vi "Return Msg.vi"(8 "error in (no error)":errorcluster, 11 "Add Control_Behavior.lvclass":refnum<class "Add Control_Behavior.lvclass">) -> (0 "error out":errorcluster, 2 "Console Reply.lvclass":refnum<class "Console Reply.lvclass">, 3 "Panel Behavior.lvclass":refnum<class "Panel Behavior.lvclass">)   [LabVIEW 2015, in "Add Control_Behavior.lvclass"]
uses:
  Add Control_Behavior.lvclass
  _Depences/Panel API/Panel Request/Panle Requeset Behavior/Panel Behavior.lvclass
  _Depences/Panel API/Console Reply/Console Reply/Console Reply.lvclass
  Console Reply Add Control Result/Console Reply Add Control.lvclass
  Add Control_Behavior.lvclass/Add Control_Behavior.ctl
  Console Reply Add Control Result/Console Reply Add Control.lvclass/Console Reply Add Control.ctl
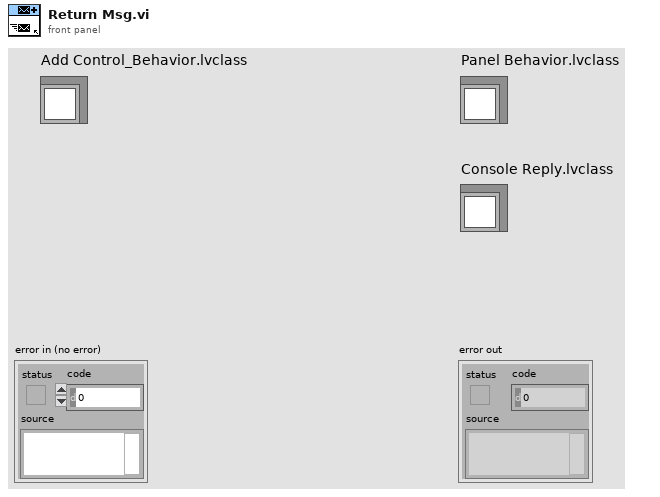
[diagram p1: front panel]
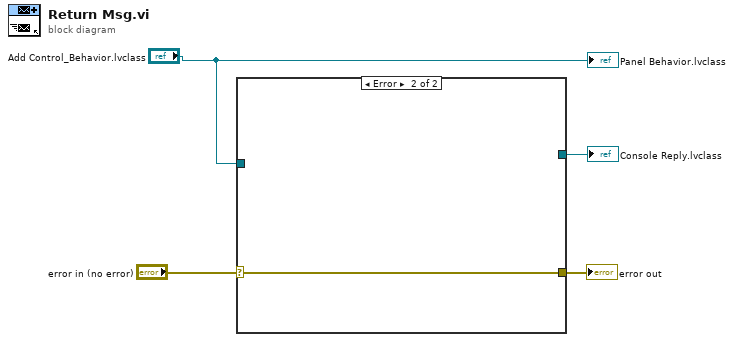
[diagram p0: block diagram]
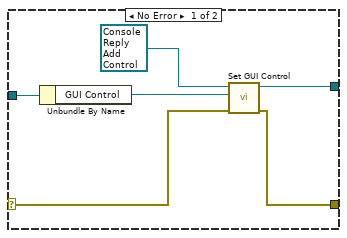
[diagram p2: hidden frame]
diagram:
  n1 = case shown="Error" "error in (no error)" {
    selector: "error in (no error)" -> [w6 w11]
    tunnel: "Add Control_Behavior.lvclass" -> [w10 _]
    tunnel: [w7 _] -> w3
    tunnel: [w5 w11] -> w1
    frame No Error {
      n2 = Unbundle By Name(w10) -> ("GUI Control"=w8:refnum<class "GUI Control.lvclass">)
      n3 = call "Set GUI Control.vi"("error in (no error)"=w6, "GUI Control"=w8, "Console Reply Add Control in"=refnum<class "Console Reply Add Control.lvclass"> refnum) -> ("error out"=w5:errorcluster, "Console Reply Add Control out"=w7:refnum<class "Console Reply Add Control.lvclass">)  [unwired: 7 in]
    }
    frame Error {
    }
  }
  "error out" <- w1
  "Console Reply.lvclass" <- w3
  "Panel Behavior.lvclass" <- "Add Control_Behavior.lvclass"
